vi "TestSpaceshipMove.vi"() -> ()   [LabVIEW 2017]
uses:
  Display/Display_mods.ctl
  Spaceship/Spaceship_mods.ctl
  ManageMovableObjects/ManRef_mods.ctl
  <vilib>/Utility/inputDevices.llb/keyboardAcquire.vi
  <vilib>/Utility/inputDevices.llb/closeKeyboard.vi
panel:
  out "error out":errorcluster
  in  "stop":bool
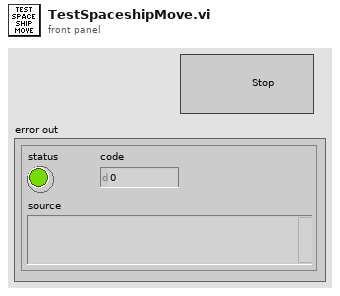
[diagram p1: front panel]
types:
  T1 = typedef "Display_mods.ctl" = enum16{"Init", "GetBase", "AddAster", "UpdateShip", "AddShoot", "DrawAll", "Clear", "Close"}
  T2 = typedef "ManRef_mods.ctl" = enum16{"Init", "NewAster", "MoveAll", "DestroyAster", "NewShoot", "DestroyShot", "CheckColision", "End"}
  T3 = typedef "Spaceship_mods.ctl" = enum16{"Init", "Move", "Rotate", "Translate", "GetData", "End"}
  T4 = enum16{"0", "1", "2", "3", "4", "5", "6", "7", "8", "9", "A", "B", "C", "D", "E", "F", "G", "H", "I", "J", "K", "L", "M", "N", "O", "P", "Q", "R", "S", "T", "U", "V", "W", "X", "Y", "Z", "F1", "F2", "F3", "F4", "F5", "F6", "F7", "F8", "F9", "F10", "F11", "F12", "F13", "F14", "F15", "ADD", "BACK", "BACKSLASH", "CAPITAL", "COMMA", "DECIMAL", "DELETE", "DIVIDE", "DOWN", "END", "EQUALS", "ESCAPE", "GRAVE (`)", "HOME", "INSERT", "LBRACKET", "LCONTROL", "LEFT", "L ALT", "LSHIFT", "LWIN", "MINUS", "MULTIPLY", "NEXT", "NUMLOCK", "NUMPAD_0", "NUMPAD_1", "NUMPAD_2", "NUMPAD_3", "NUMPAD_4", "NUMPAD_5", "NUMPAD_6", "NUMPAD_7", "NUMPAD_8", "NUMPAD_9", "PAUSE", "PERIOD", "PRIOR (PG UP)", "RBRACKET", "RCONTROL", "RETURN", "RIGHT", "R ALT", "RSHIFT", "RWIN", "SCROLL", "SEMICOLON", "SLASH", "SPACE", "SUBTRACT", "TAB", "UP", "ENTER (num pad)", "' (quote)"}[]
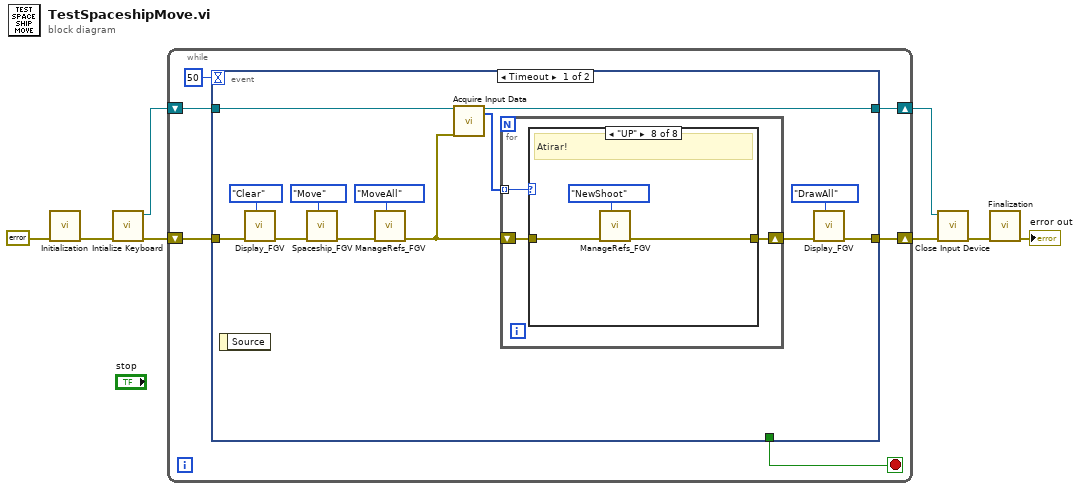
[diagram p0: block diagram]
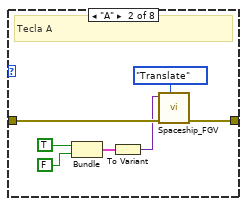
[diagram p3: hidden frame]
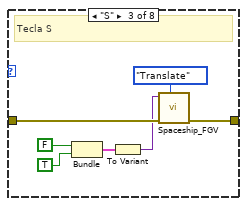
[diagram p4: hidden frame]
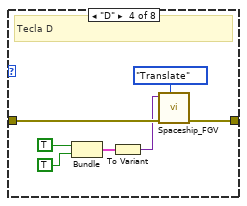
[diagram p5: hidden frame]
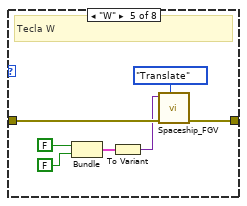
[diagram p6: hidden frame]
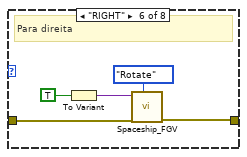
[diagram p7: hidden frame]
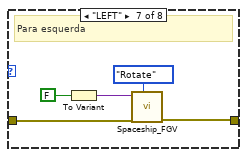
[diagram p8: hidden frame]
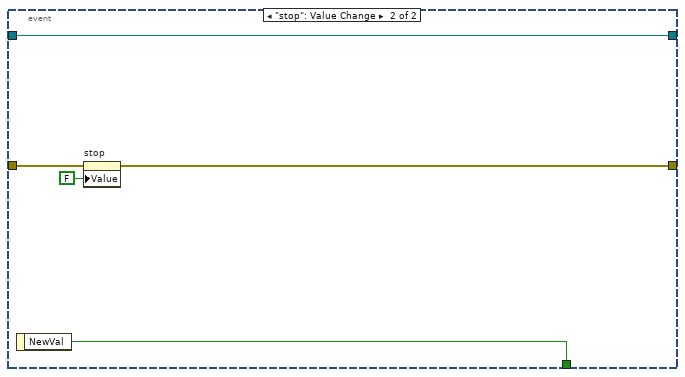
[diagram p9: hidden frame]
diagram:
  n1 = call "Initialization.vi"("error in"=errorcluster {"status"=FALSE, "code"=0, "source"=""}) -> ("error out"=w6:errorcluster)  [unwired: 10 in]
  n2 = call <vilib>:"Intialize Keyboard.vi"("error in (no error)"=w6) -> ("error out"=w5:errorcluster, "device ID"=w4:refnum<k1>)  [unwired: 9 in]
  n3 = while {
    shift-right: [w13] -> w3
    shift-left: w5 -> [w14]
    shift-right: [w9] -> w1
    shift-left: w4 -> [w10]
    stop <- w11 stop-if-true
    n4 = event shown="[0] Timeout" {
      selector: _ -> [_ _]
      dyn-events: _ -> [_ _]
      timeout: 50 -> [_ _]
      tunnel: w14 -> [w26 w75]
      tunnel: [w15 w74] -> w13
      tunnel: [_ w77] -> w11
      tunnel: w10 -> [w23 w73]
      tunnel: [w22 w73] -> w9
      event Timeout {
        n5 = event-data() -> ()  [unwired: 1 in, 1 out]
        n6 = call "Display_FGV.vi"("Display_mods"=Display_mods."Clear", "error in"=w26) -> ("error out"=w25:errorcluster)  [unwired: 8 in, 1 out]
        n7 = call "Spaceship_FGV.vi"("Spaceship_mods"=Spaceship_mods."Move", "error in"=w25) -> ("error out"=w20:errorcluster)  [unwired: 8 in, 1 out]
        n8 = call "ManageRefs_FGV.vi"("ManRef_mods"=ManRef_mods."MoveAll", "error in"=w20) -> ("error out"=w18:errorcluster)  [unwired: 8 in, 1 out]
        n9 = call-poly <vilib>:"Acquire Input Data.vi"("device ID"=w23, "error in (no error)"=w18) -> ("device ID"=w22:refnum<k1>, "keys pressed"=w21:T4)  [unwired: 15 in, 1 out]
        n10 = for {
          shift-right: [w29] -> w16
          shift-left: w18 -> [w30]
          tunnel: w21 -> [w28] mode=indexing
          n11 = case shown="\"UP\"" w28 {
            tunnel: w30 -> [w31 w37 w44 w51 w58 w63 w68 w71]
            tunnel: [w31 w36 w43 w50 w57 w62 w67 w70] -> w29
            frame "0", Default {
            }
            frame "A" {
              # "Tecla A"
              n12 = Bundle("stop"=TRUE, "stop"=FALSE) -> (w35:cluster{"stop":bool, "stop":bool})  [unwired: 1 in]
              n13 = To Variant(anything=w35) -> (Variant=w34:variant)
              n14 = call "Spaceship_FGV.vi"("Spaceship_mods"=Spaceship_mods."Translate", "error in"=w37, "DataIn"=w34) -> ("error out"=w36:errorcluster)  [unwired: 7 in, 1 out]
            }
            frame "S" {
              # "Tecla S"
              n15 = Bundle("stop"=FALSE, "stop"=TRUE) -> (w42:cluster{"stop":bool, "stop":bool})  [unwired: 1 in]
              n16 = To Variant(anything=w42) -> (Variant=w41:variant)
              n17 = call "Spaceship_FGV.vi"("Spaceship_mods"=Spaceship_mods."Translate", "error in"=w44, "DataIn"=w41) -> ("error out"=w43:errorcluster)  [unwired: 7 in, 1 out]
            }
            frame "D" {
              # "Tecla D"
              n18 = Bundle("stop"=TRUE, "stop"=TRUE) -> (w49:cluster{"stop":bool, "stop":bool})  [unwired: 1 in]
              n19 = To Variant(anything=w49) -> (Variant=w48:variant)
              n20 = call "Spaceship_FGV.vi"("Spaceship_mods"=Spaceship_mods."Translate", "error in"=w51, "DataIn"=w48) -> ("error out"=w50:errorcluster)  [unwired: 7 in, 1 out]
            }
            frame "W" {
              # "Tecla W"
              n21 = Bundle("stop"=FALSE, "stop"=FALSE) -> (w56:cluster{"stop":bool, "stop":bool})  [unwired: 1 in]
              n22 = To Variant(anything=w56) -> (Variant=w55:variant)
              n23 = call "Spaceship_FGV.vi"("Spaceship_mods"=Spaceship_mods."Translate", "error in"=w58, "DataIn"=w55) -> ("error out"=w57:errorcluster)  [unwired: 7 in, 1 out]
            }
            frame "RIGHT" {
              # "Para direita"
              n24 = To Variant(anything=TRUE ("stop")) -> (Variant=w61:variant)
              n25 = call "Spaceship_FGV.vi"("Spaceship_mods"=Spaceship_mods."Rotate", "error in"=w63, "DataIn"=w61) -> ("error out"=w62:errorcluster)  [unwired: 7 in, 1 out]
            }
            frame "LEFT" {
              # "Para esquerda"
              n26 = To Variant(anything=FALSE ("stop")) -> (Variant=w66:variant)
              n27 = call "Spaceship_FGV.vi"("Spaceship_mods"=Spaceship_mods."Rotate", "error in"=w68, "DataIn"=w66) -> ("error out"=w67:errorcluster)  [unwired: 7 in, 1 out]
            }
            frame "UP" {
              # "Atirar!"
              n28 = call "ManageRefs_FGV.vi"("ManRef_mods"=ManRef_mods."NewShoot", "error in"=w71) -> ("error out"=w70:errorcluster)  [unwired: 8 in, 1 out]
            }
          }
        }
        n29 = call "Display_FGV.vi"("Display_mods"=Display_mods."DrawAll", "error in"=w16) -> ("error out"=w15:errorcluster)  [unwired: 8 in, 1 out]
      }
      event "stop": Value Change {
        n30 = event-data() -> ("NewVal"=w77:bool)  [unwired: 1 in]
        n31 = property on="stop" class="Bool (strict)"(error in=w75, "Value"=FALSE ("Add")) -> (error out=w74:errorcluster)  [unwired: 1 in, 1 out]
      }
    }
  }
  n32 = call-poly <vilib>:"Close Input Device.vi"("error in (no error)"=w3, "device ID"=w1) -> ("error out"=w2:errorcluster)  [unwired: 8 in]
  n33 = call "Finalization.vi"("error in"=w2) -> ("error out"=→"error out":errorcluster)  [unwired: 10 in]
